vi "海伦公式.vi"(7 "A":dbl, 10 "C":dbl, 11 "B":dbl) -> (3 "S":dbl)   [LabVIEW 2018]
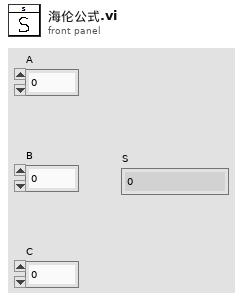
[diagram p1: front panel]
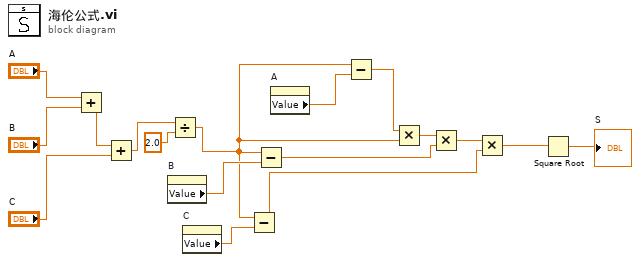
[diagram p0: block diagram]
diagram:
  n1 = Add(x="A", y="B") -> (x+y=w14:dbl)
  n2 = Add(x=w14, y="C") -> (x+y=w3:dbl)
  n3 = property on="B" class="DigNum (严格)"() -> ("Value"=w12:dbl)  [unwired: 2 in, 2 out]
  n4 = Divide(x=w3, y=2.0) -> (x/y=w1:dbl)
  n5 = property on="C" class="DigNum (严格)"() -> ("Value"=w11:dbl)  [unwired: 2 in, 2 out]
  n6 = Subtract(x=w1, y=w11) -> (x-y=w6:dbl)
  n7 = Subtract(x=w1, y=w12) -> (x-y=w8:dbl)
  n8 = property on="A" class="DigNum (严格)"() -> ("Value"=w13:dbl)  [unwired: 2 in, 2 out]
  n9 = Subtract(x=w1, y=w13) -> (x-y=w10:dbl)
  n10 = Multiply(x=w10, y=w1) -> (x*y=w9:dbl)
  n11 = Multiply(x=w9, y=w8) -> (x*y=w7:dbl)
  n12 = Multiply(x=w7, y=w6) -> (x*y=w5:dbl)
  n13 = Square Root(x=w5) -> (sqrt(x)=→"S":dbl)
